vi "Generate Move2Position Command.vi"(8 "error in (no error)":errorcluster, 9 "Pos.Z(um)":string, 10 "Pos.Y(um)":string, 11 "Pos.X(um)":string) -> (0 "error out":errorcluster, 3 "Move2Position Command OUT":string)   [LabVIEW 2012]
doc: "SciScan 1.2 160622"
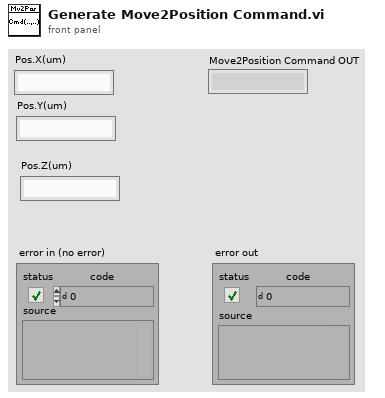
[diagram p1: front panel]
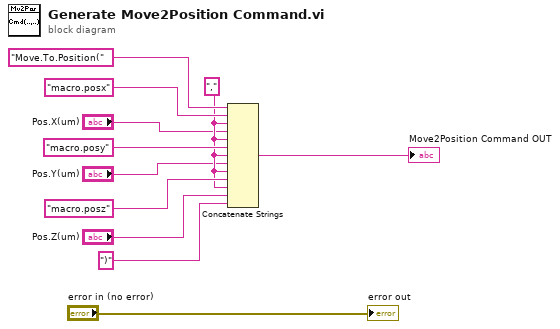
[diagram p0: block diagram]
diagram:
  w7 = "," ("Variable Name in")
  n1 = Concatenate Strings("Move.To.Position(" ("Variable Name in"), "macro.posx" ("Variable Name in"), w7, "Pos.X(um)", w7, "macro.posy" ("Variable Name in"), w7, "Pos.Y(um)", w7, "macro.posz" ("Variable Name in"), w7, "Pos.Z(um)", ")" ("string")) -> (→"Move2Position Command OUT":string)
  "error out" <- "error in (no error)"
